vi "Temp ctrl - Setpoint.vi"(8 "Error In":errorcluster, 10 "Setpoint":dbl[unit], 11 "Temp handle":T1={"Connected"=FALSE, "Temp ctrl"={"Gain (P)"=0.0, "Reset (I)"=0.0, "Rate (D)"=0, "Stabilization rate"=0.0, "Stabilization delta"=0.0, "Type"=enum."Lake Shore 325", "Custom temp ctrl"={"VISA resource name"=""}, "Lakeshore 325"={"VISA name"="", "Loop"=0, "Heater Range"=1, "Heater Resistance"=0, "Sample sensor"=0, "Fast sensor"=0, "Slow sensor"=0}}} {"Temp ctrl"."Lakeshore 325"."Slow sensor" items=["A", "B"]; "Temp ctrl"."Lakeshore 325"."Fast sensor" items=["A", "B"]; "Temp ctrl"."Lakeshore 325"."Sample sensor" items=["A", "B"]; "Temp ctrl"."Lakeshore 325"."Heater Resistance" items=["25 Ohm"=1, "50 Ohm"=2]; "Temp ctrl"."Lakeshore 325"."Heater Range" items=["Off", "Low (loop 1) or On (loop 2)", "High (loop 1)"]; "Temp ctrl"."Lakeshore 325"."Loop" items=["Loop 1"=1, "Loop 2"=2]}) -> (0 "Error Out":errorcluster)   [LabVIEW 2019]
doc: "Applies temperature setpoint to a temperature controller"
uses:
  Type defs/Temp handle Type Def.ctl
  Type defs/Temp ctrl Type Def.ctl
  Custom devices/Custom temp ctrl settings.ctl
  <instrlib>/Lake Shore 325/Lake Shore 325.lvlib
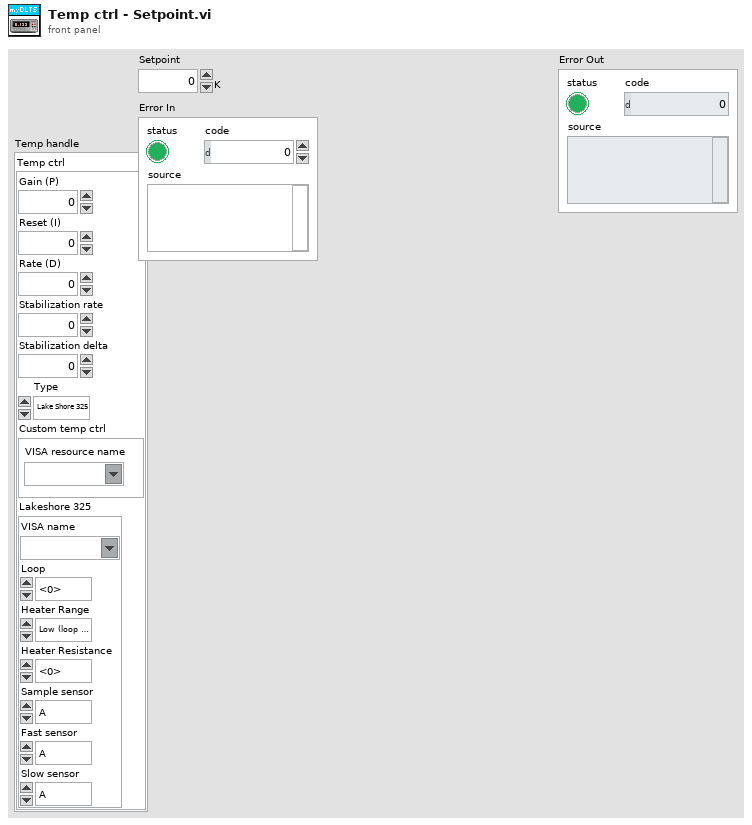
[diagram p1: front panel]
types:
  T1 = typedef "Temp handle Type Def.ctl" = cluster{"Connected":bool, "Temp ctrl":T2}
  T2 = typedef "Temp ctrl Type Def.ctl" = cluster{"Gain (P)":dbl, "Reset (I)":dbl, "Rate (D)":u16, "Stabilization rate":dbl, "Stabilization delta":dbl, "Type":enum16{"Custom", "Lake Shore 325"}, "Custom temp ctrl":T3, "Lakeshore 325":cluster{"VISA name":refnum<visa-resource-name>, "Loop":u16, "Heater Range":u16, "Heater Resistance":u16, "Sample sensor":u16, "Fast sensor":u16, "Slow sensor":u16}}
  T3 = typedef "Custom temp ctrl settings.ctl" = cluster{"VISA resource name":refnum<visa-resource-name>}
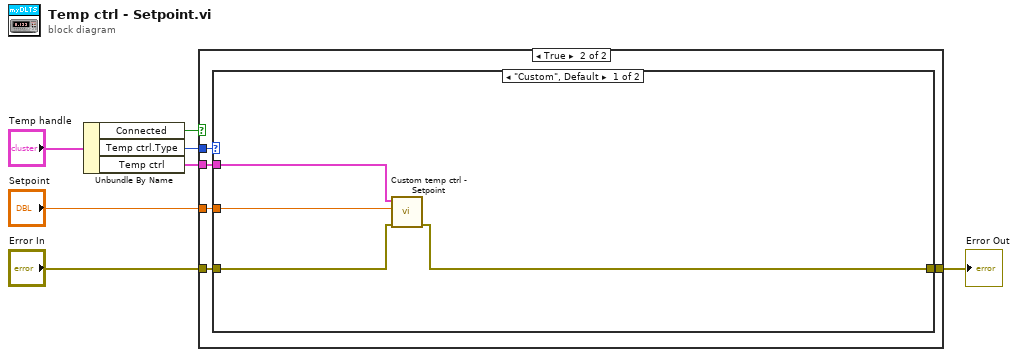
[diagram p0: block diagram]
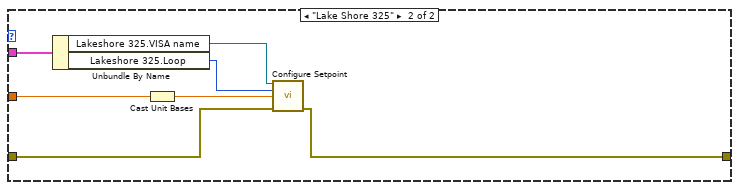
[diagram p3: hidden frame]
diagram:
  n1 = Unbundle By Name("Temp handle") -> ("Connected"=w7:bool, "Temp ctrl.Type"=w6:enum16{"Custom", "Lake Shore 325"}, "Temp ctrl"=w4:T2)
  n2 = case shown="True" w7 {
    tunnel: w6 -> [_ w13]
    tunnel: w4 -> [_ w12]
    tunnel: "Setpoint" -> [_ w11]
    tunnel: "Error In" -> [w8 w10]
    tunnel: [w8 w9] -> w1
    frame False {
    }
    frame True {
      n3 = case shown="\"Custom\", Default" w13 {
        tunnel: w12 -> [w17 w24]
        tunnel: w11 -> [w16 w22]
        tunnel: w10 -> [w15 w23]
        tunnel: [w14 w18] -> w9
        frame "Custom", Default {
          n4 = call "Custom temp ctrl - Setpoint.vi"("Error In"=w15, "Setpoint"=w16, "Temp ctrl"=w17) -> ("Error Out"=w14:errorcluster)  [unwired: 8 in]
        }
        frame "Lake Shore 325" {
          n5 = Unbundle By Name(w24) -> ("Lakeshore 325.VISA name"=w20:refnum<visa-resource-name>, "Lakeshore 325.Loop"=w19:u16)
          n6 = Cast Unit Bases(0:w22) -> (2:w21:dbl)  [unwired: 1 in]
          n7 = call <instrlib>:"Configure Setpoint.vi"("VISA resource name"=w20, "Loop (1:Loop 1)"=w19, "Setpoint Value (0.0000)"=w21, "error in (no error)"=w23) -> ("error out"=w18:errorcluster)  [unwired: 10 in, 1 out]
        }
      }
    }
  }
  "Error Out" <- w1
